vi "Write Local Msg Set.vi"(11 "TEMPLATE Actor in":refnum<class "TEMPLATE Actor.lvclass">) -> (3 "TEMPLATE Actor out":refnum<class "TEMPLATE Actor.lvclass">)   [LabVIEW 2025, in "TEMPLATE Actor.lvlib" / "TEMPLATE Actor.lvclass"]
uses:
  TEMPLATE Actor.lvclass
  TEMPLATE Actor.lvclass/TEMPLATE Actor.ctl
  <vilib>/Nathan Davis/jettl/jettl/jettl/Actor/Actor/Actor.lvclass
  <vilib>/Nathan Davis/jettl/jettl/jettl/Actor/Actor.lvlib
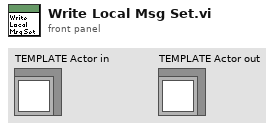
[diagram p1: front panel]
types:
  T1 = typedef "jettl.lvlib/Actor.lvlib/Msg Set.ctl" = set{refnum<class "Msg.lvclass">}
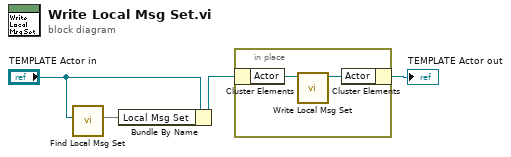
[diagram p0: block diagram]
diagram:
  n1 = call <vilib>:"Find Local Msg Set.vi"("Variant (X Actor.lvclass)"="TEMPLATE Actor in") -> ("Local Msg Set"=w1:T1)  [unwired: 10 in]
  n2 = Bundle By Name(cluster="TEMPLATE Actor in", "Local Msg Set"=w1) -> (w3:refnum<class "TEMPLATE Actor.lvclass">)
  n3 = in-place {
    n4 = in-place-cluster #1(w3) -> ("Actor"=w6:refnum<class "Actor.lvclass">)
    n5 = call-dynamic "Write Local Msg Set.vi"("Actor in"=w6) -> ("Actor out"=w5:refnum<class "Actor.lvclass">)  [unwired: 10 in]
    n6 = in-place-cluster #1("Actor"=w5) -> (→"TEMPLATE Actor out":refnum<class "TEMPLATE Actor.lvclass">)
  }
